vi "BITMAPINFOHEADER.vi"(11 "图像维数":i32[](array[numeric])) -> (3 "位图文件头":u8[](array[numeric]))   [LabVIEW 2012]
panel:
  out "大小":i32
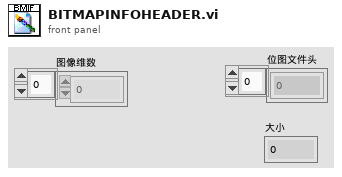
[diagram p1: front panel]
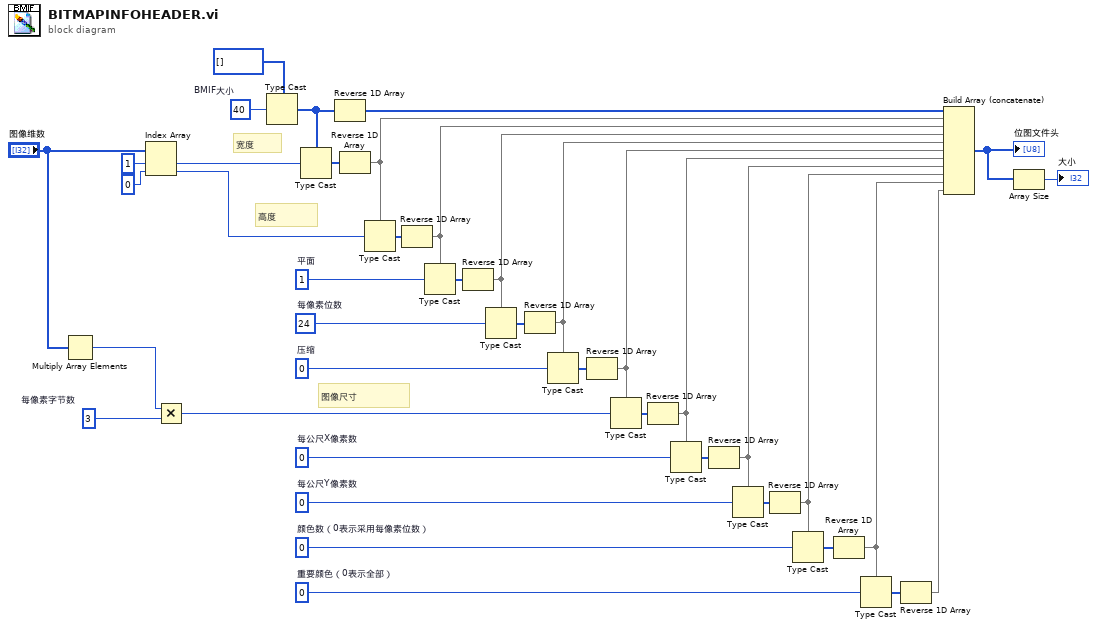
[diagram p0: block diagram]
diagram:
  w26 = 3  # 每像素字节数
  w29 = 0  # 重要颜色（0表示全部）
  w30 = 0  # 颜色数（0表示采用每像素位数）
  w33 = 0  # 每公尺Y像素数
  w34 = 0  # 每公尺X像素数
  w35 = 0  # 压缩
  w36 = i16 24  # 每像素位数
  w37 = i16 1  # 平面
  w38 = 40  # BMIF大小
  # "图像尺寸"
  # "高度"
  # "宽度"
  n1 = Multiply Array Elements ("数组元素相乘")(1:"图像维数") -> (0:w2:i32)
  n2 = Index Array ("索引数组")(array="图像维数", index #1=1 ("索引"), index #2=0 ("索引")) -> (element #1=w27:i32, element #2=w28:i32)
  n3 = Multiply ("乘")(x=w2, y=w26) -> (x*y=w1:i32)
  n4 = Type Cast ("强制类型转换")(type=u8[] [], x=w38) -> (*(type *) &x=w7:u8[])
  n5 = Type Cast ("强制类型转换")(type=w7, x=w27) -> (*(type *) &x=w25:u8[])
  n6 = Reverse 1D Array ("反转一维数组")(array=w7) -> (reversed array=w6:u8[])
  n7 = Reverse 1D Array ("反转一维数组")(array=w25) -> (reversed array=w24:u8[])
  n8 = Type Cast ("强制类型转换")(type=w24, x=w28) -> (*(type *) &x=w23:u8[])
  n9 = Reverse 1D Array ("反转一维数组")(array=w23) -> (reversed array=w22:u8[])
  n10 = Type Cast ("强制类型转换")(type=w22, x=w37) -> (*(type *) &x=w21:u8[])
  n11 = Reverse 1D Array ("反转一维数组")(array=w21) -> (reversed array=w20:u8[])
  n12 = Type Cast ("强制类型转换")(type=w20, x=w36) -> (*(type *) &x=w19:u8[])
  n13 = Reverse 1D Array ("反转一维数组")(array=w19) -> (reversed array=w18:u8[])
  n14 = Type Cast ("强制类型转换")(type=w18, x=w35) -> (*(type *) &x=w17:u8[])
  n15 = Reverse 1D Array ("反转一维数组")(array=w17) -> (reversed array=w16:u8[])
  n16 = Type Cast ("强制类型转换")(type=w16, x=w1) -> (*(type *) &x=w15:u8[])
  n17 = Reverse 1D Array ("反转一维数组")(array=w15) -> (reversed array=w14:u8[])
  n18 = Type Cast ("强制类型转换")(type=w14, x=w34) -> (*(type *) &x=w13:u8[])
  n19 = Reverse 1D Array ("反转一维数组")(array=w13) -> (reversed array=w12:u8[])
  n20 = Type Cast ("强制类型转换")(type=w12, x=w33) -> (*(type *) &x=w11:u8[])
  n21 = Reverse 1D Array ("反转一维数组")(array=w11) -> (reversed array=w10:u8[])
  n22 = Type Cast ("强制类型转换")(type=w10, x=w30) -> (*(type *) &x=w9:u8[])
  n23 = Reverse 1D Array ("反转一维数组")(array=w9) -> (reversed array=w8:u8[])
  n24 = Type Cast ("强制类型转换")(type=w8, x=w29) -> (*(type *) &x=w5:u8[])
  n25 = Reverse 1D Array ("反转一维数组")(array=w5) -> (reversed array=w4:u8[])
  n26 = Build Array (concatenate) ("创建数组")(w6, w24, w22, w20, w18, w16, w14, w12, w10, w8, w4) -> (w32:u8[])
  "位图文件头" <- w32
  n27 = Array Size ("数组大小")(array=w32) -> (size(s)=→"大小":i32)
